vi "PICTURE _LOad to Reference.vi"(0 "Path":path, 5 "error -IN":errorcluster, 6 "ImagePaths":string[](array[string])=["IMAGES\\Company.gif", "IMAGES\\Division.gif", "IMAGES\\Contact.gif"]) -> (15 "PicRefs":refnum<k7>[](array[refnum]), 17 "Array":string[](array[string]), 19 "error OUT":errorcluster)   [LabVIEW 2019]
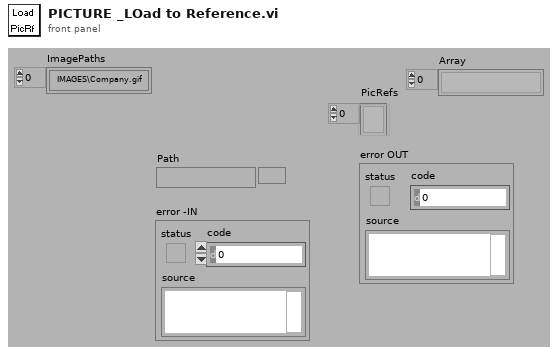
[diagram p1: front panel]
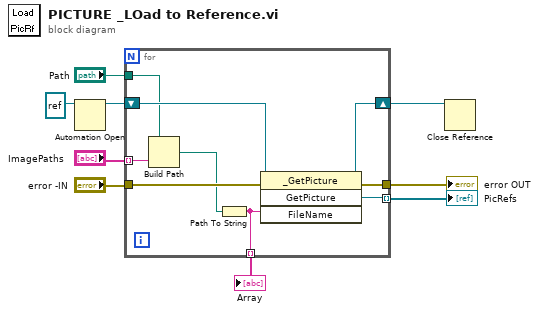
[diagram p0: block diagram]
diagram:
  n1 = Automation Open(Automation Refnum=refnum<k7> refnum ("PicRef -IN")) -> (Automation Refnum=w6:refnum<k7>)  [unwired: 2 in, 2 out]
  n2 = for {
    tunnel: [w17] -> w8 mode=indexing
    shift-right: [w14] -> w5
    shift-left: w6 -> [w15]
    tunnel: "ImagePaths" -> [w13] mode=indexing
    tunnel: "Path" -> [w11]
    tunnel: "error -IN" -> [w18]
    tunnel: [w16] -> w7
    tunnel: [w10] -> w1 mode=indexing
    n3 = Build Path(base path=w11, name or relative path=w13) -> (appended path=w12:path)
    n4 = Path To String(path=w12) -> (string=w10:string)
    n5 = invoke class="_GetPicture" method="GetPicture"(reference=w15, error in=w18, "FileName"=w10) -> (reference out=w14:refnum<k7>, error out=w16:errorcluster, "GetPicture"=w17:refnum<k7>)  [unwired: 1 in, 1 out]
  }
  "PicRefs" <- w8
  "error OUT" <- w7
  "Array" <- w1
  n6 = Close Reference(reference=w5) -> ()  [unwired: 1 in, 1 out]
